vi "Teleop.vi"(6 "error in (no error)":errorcluster, 8 "Match Info":T1={"Autonomous Elapsed Seconds"=0.0, "TeleOp Elapsed Seconds"=0.0, "Disabled Elapsed Seconds"=0.0, "Visited Autonomous"=FALSE, "Visited TeleOp"=FALSE, "Visited Disabled"=FALSE, "Autonomous Settings"={"Autonomous Style"=enum."Independent", "VI Refnum"=refnum}}, 9 "Call Context":T2) -> (0 "error out":errorcluster, 1 "Throttle":dbl, 2 "Motors":dbl[](array[slide]) scale=-1.0..1.0)   [LabVIEW 2013]
doc: "This VI is called for each TeleOp packet received from the DS where the robot is not disabled. It is often used to read from the joysticks and update I/O or to update setpoints for timed control loops. It should complete and return within 20 milliseconds or it may miss DS packets."
uses:
  <vilib>/Rock Robotics/WPI/DriverStation/WPI_DriverStationDerivedRobotMode.ctl
  <vilib>/Rock Robotics/WPI/DriverStation/WPI_DriverStationMatch Info.ctl
  <vilib>/Rock Robotics/WPI/Relay/WPI_RelayValue.ctl
  Robot Global Data.vi
  <vilib>/Rock Robotics/WPI/RobotDrive/WPI_RobotDriveArcadeDrive_Standard(NoSaturation).vi
  <vilib>/Rock Robotics/WPI/Joystick/WPI_JoystickGetSetRefNum.vi
  <vilib>/Rock Robotics/WPI/RobotDrive/WPI_RobotDriveGetSetRefNum.vi
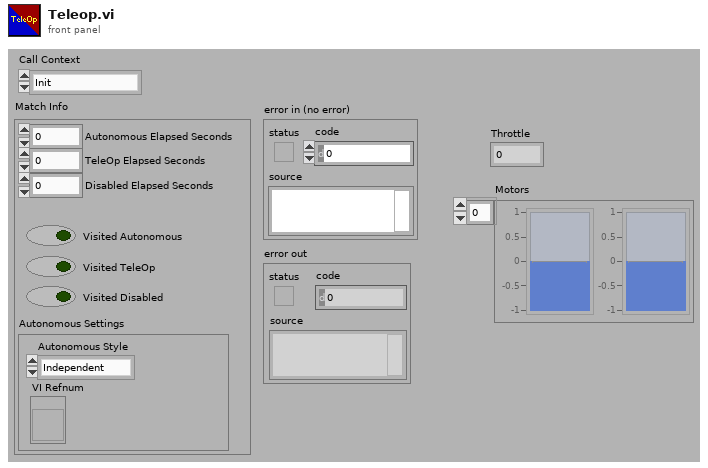
[diagram p1: front panel]
types:
  T1 = typedef "WPI_DriverStationMatch Info.ctl" = cluster{"Autonomous Elapsed Seconds":dbl, "TeleOp Elapsed Seconds":dbl, "Disabled Elapsed Seconds":dbl, "Visited Autonomous":bool, "Visited TeleOp":bool, "Visited Disabled":bool, "Autonomous Settings":cluster{"Autonomous Style":enum16{"Iterative", "Independent"}, "VI Refnum":refnum<vi>}}
  T2 = typedef "WPI_DriverStationDerivedRobotMode.ctl" = enum16{"Init", "Execute", "Stop"}
  T3 = typedef "WPI_JoystickDevRef.ctl" = cluster{"Device":T4}
  T4 = typedef "WPI_JoystickDeviceEnum.ctl" = enum16{"USB 1", "USB 2", "USB 3", "USB 4", "Kinect 1", "Kinect 2"}
  T5 = typedef "WPI_JoystickButtonState.ctl" = cluster{"Button 1":bool, "Button 2":bool, "Button 3":bool, "Button 4":bool, "Button 5":bool, "Button 6":bool, "Button 7":bool, "Button 8":bool, "Button 9":bool, "Button 10":bool, "Button 11":bool, "Button 12":bool}
  T6 = cluster{"axis 1 (x)":dbl, "axis 2 (y)":dbl, "axis 3 (throttle)":dbl, "axis 4":dbl, "axis 5":dbl, "axis 6":dbl}
  T7 = typedef "WPI_RelayValue.ctl" = enum16{"Off", "On", "Forward", "Reverse"}
  T8 = typedef "WPI_RobotDriveDevRef.ctl" = cluster{"DevStatus":errorcluster, "Motors[]":T9[], "Square Inputs":bool, "Max Output":dbl, "Isochronous":bool}
  T9 = typedef "WPI_MotorControlDeviceRef.ctl" = cluster{"DeviceStatus":errorcluster, "Type":enum16{"PWM", "CAN"}, "PWM":cluster{"Digital Module":T10, "PWM Channel":T11, "DeadBand":T12}, "CAN":cluster{"Device Number":u8, "Control Mode":T13, "Semaphore":T14, "Max Vout":dbl}, "Invert":bool, "TransformRef":T15, "InvTransformRef":T15}
  T10 = typedef "FPGA_TypedefDigitalModule.ctl" = enum16{"Digital Module 1", "Digital Module 2"}
  T11 = typedef "FPGA_DIOPWMChannel.ctl" = enum8{"PWM 1", "PWM 2", "PWM 3", "PWM 4", "PWM 5", "PWM 6", "PWM 7", "PWM 8", "PWM 9", "PWM 10", "Invalid"}
  T12 = typedef "WPI_PWMDeadband.ctl" = cluster{"Name":string, "maxPositivePwm":i32, "minPositivePwm":i32, "centerPwm":i32, "maxNegativePwm":i32, "minNegativePwm":i32, "angularRange":u16}
  T13 = typedef "WPI_CANJaguar_ControlMode.ctl" = enum8{"Percent VBus", "Current", "Speed", "Position", "Voltage"}
  T14 = typedef "Semaphore RefNum" = refnum<k1>
  T15 = typedef "WPI_PWMTransform_ConPane.ctl" = refnum<vi>
  T16 = typedef "WPI_RelayDevRef.ctl" = cluster{"DevStatus":errorcluster, "Relay Channel":T17, "Digital Module":T10, "Relay Direction":T18}
  T17 = typedef "FPGA_DIORelayChannel.ctl" = enum8{"Relay 1", "Relay 2", "Relay 3", "Relay 4", "Relay 5", "Relay 6", "Relay 7", "Relay 8", "Invalid"}
  T18 = typedef "WPI_RelayDirection.ctl" = enum16{"Both directions", "Forward only", "Reverse only"}
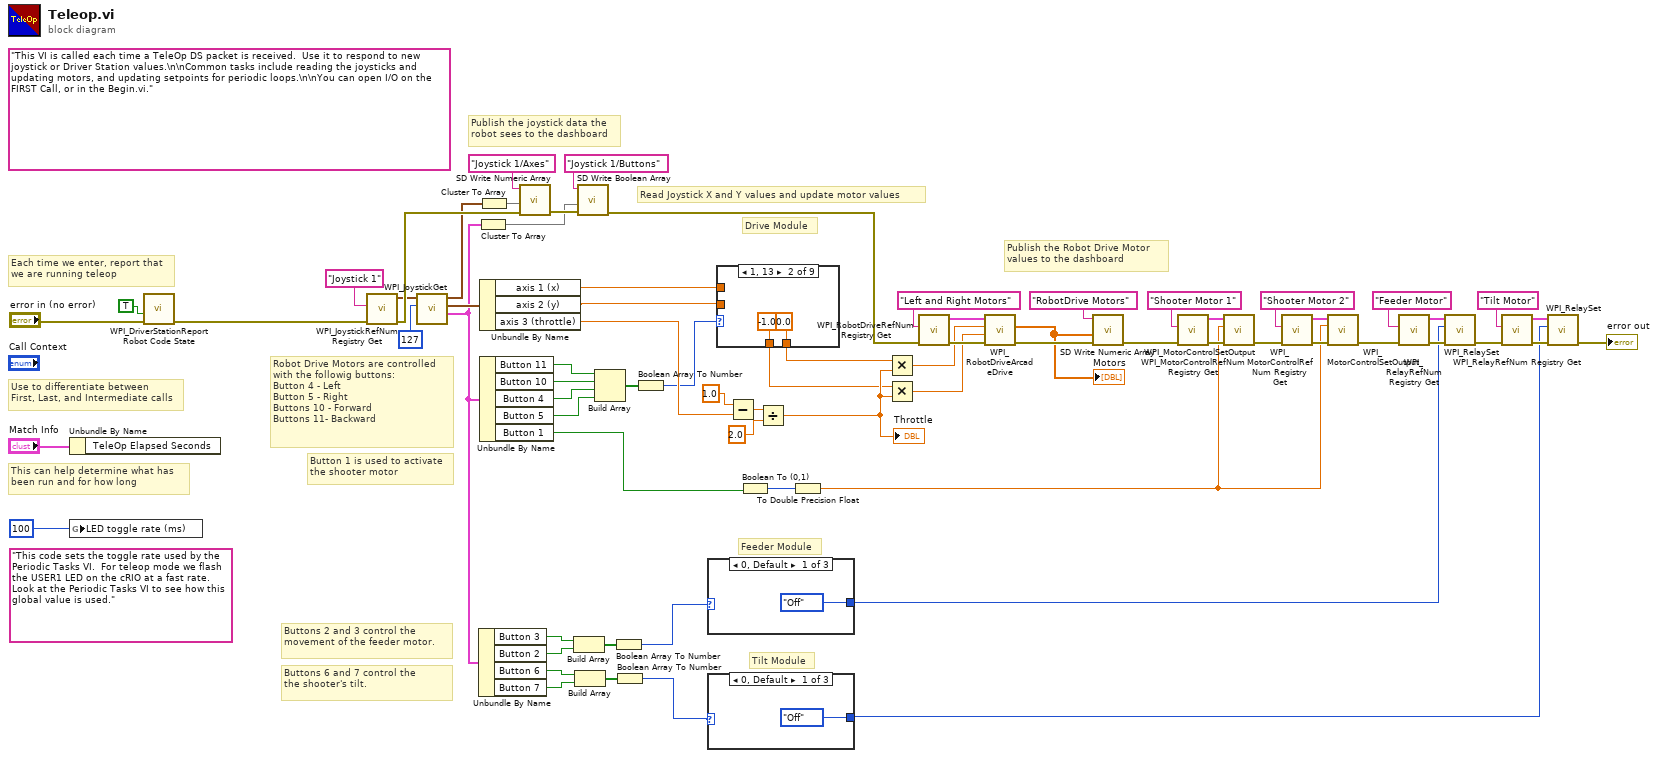
[diagram p0: block diagram]
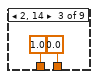
[diagram p3: hidden frame]
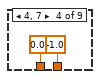
[diagram p4: hidden frame]
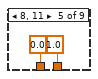
[diagram p5: hidden frame]
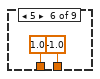
[diagram p6: hidden frame]
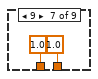
[diagram p7: hidden frame]
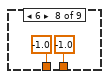
[diagram p8: hidden frame]
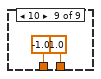
[diagram p9: hidden frame]
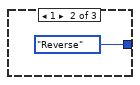
[diagram p10: hidden frame]
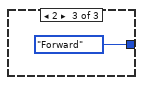
[diagram p11: hidden frame]
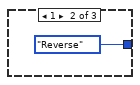
[diagram p12: hidden frame]
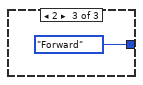
[diagram p13: hidden frame]
diagram:
  (unwired) "This code sets the toggle rate used by the Periodic Tasks VI.  For teleop mode we flash the USER1 LED on the cRIO at a fast rate.  Look at the Periodic Tasks VI to see how this global value is used."
  (unwired) "This VI is called each time a TeleOp DS packet is received.  Use it to respond to new joystick or Driver Station values.\n\nCommon tasks include reading the joysticks and updating motors, and updating setpoints for periodic loops.\n\nYou can open I/O on the FIRST Call, or in the Begin.vi."
  # "Buttons 6 and 7 control the\nthe shooter's tilt."
  # "Buttons 2 and 3 control the\nmovement of the feeder motor."
  # "Feeder Module"
  # "Tilt Module"
  # "Drive Module"
  # "Robot Drive Motors are controlled\nwith the followig buttons:\nButton 4 - Left\nButton 5 - Right\nButtons 10 - Forward\nButtons 11- Backward"
  # "Button 1 is used to activate\nthe shooter motor"
  # "Publish the Robot Drive Motor\nvalues to the dashboard"
  # "Read Joystick X and Y values and update motor values"
  # "Publish the joystick data the\nrobot sees to the dashboard"
  # "Each time we enter, report that\nwe are running teleop"
  # "Use to differentiate between\nFirst, Last, and Intermediate calls"
  # "This can help determine what has\nbeen run and for how long"
  n1 = Unbundle By Name("Match Info") -> ()  [unwired: 1 out]
  n2 = global write "Robot Global Data.vi" "LED toggle rate (ms)"(u32 100 ("LED ms toggle rate")) -> ()
  n3 = call <vilib>:"WPI_DriverStationReport Robot Code State.vi"("error in (no error)"="error in (no error)", "TeleOp"=TRUE ("Autonomous")) -> ("error out"=w43:errorcluster)  [unwired: 9 in]
  n4 = call <vilib>:"WPI_JoystickRefNum Registry Get.vi"("error in (no error)"=w43, "refnum name"="Joystick 1") -> ("error out"=w44:errorcluster, "JoystickDevRef"=w37:T3)  [unwired: 8 out]
  n5 = call <vilib>:"WPI_JoystickGet.vi"("Scaler"=i8 127, "JoystickDevRef"=w37) -> ("Buttons"=w34:T5, "Axes"=w51:T6, "JoystickDevRef"=w38:T3)  [unwired: 3 in]
  n6 = Cluster To Array(cluster=w34) -> (array=w39:bool[])
  n7 = Cluster To Array(cluster=w38) -> (array=w64:T4[])
  n8 = Unbundle By Name(w34) -> ("Button 3"=w20:bool, "Button 2"=w21:bool, "Button 6"=w59:bool, "Button 7"=w58:bool)
  n9 = Unbundle By Name(w51) -> ("axis 1 (x)"=w2:dbl, "axis 2 (y)"=w1:dbl, "axis 3 (throttle)"=w50:dbl)
  n10 = Unbundle By Name(w34) -> ("Button 11"=w55:bool, "Button 10"=w56:bool, "Button 4"=w36:bool, "Button 5"=w35:bool, "Button 1"=w7:bool)
  n11 = call <vilib>:"SD Write Numeric Array.vi"("error in"=w44, "Numeric Array"=w64, "Name"="Joystick 1/Axes") -> ("error out"=w42:errorcluster)  [unwired: 7 in, 1 out]
  n12 = Build Array(w20, w21) -> (w22:bool[])
  n13 = Build Array(w59, w58) -> (w57:bool[])
  n14 = call <vilib>:"SD Write Boolean Array.vi"("error in"=w42, "Boolean Array"=w39, "Name"="Joystick 1/Buttons") -> ("error out"=w41:errorcluster)  [unwired: 7 in, 1 out]
  n15 = Build Array(w55, w56, w36, w35) -> (w54:bool[])
  n16 = Boolean Array To Number(Boolean array=w22) -> (number=w19:u32)
  n17 = Boolean Array To Number(Boolean array=w57) -> (number=w11:u32)
  n18 = Boolean Array To Number(Boolean array=w54) -> (number=w3:u32)
  n19 = case shown="0, Default" w19 {
    tunnel: [WPI_RelayValue."Off" ("RelayValue") WPI_RelayValue."Reverse" ("RelayValue") WPI_RelayValue."Forward" ("RelayValue")] -> w12
    frame 0, Default {
    }
    frame 1 {
    }
    frame 2 {
    }
  }
  n20 = case shown="0, Default" w11 {
    tunnel: [WPI_RelayValue."Off" ("RelayValue") WPI_RelayValue."Reverse" ("RelayValue") WPI_RelayValue."Forward" ("RelayValue")] -> w10
    frame 0, Default {
    }
    frame 1 {
    }
    frame 2 {
    }
  }
  n21 = case shown="1, 13" w3 {
    tunnel: w2 -> [w79 _ _ _ _ _ _ _ _]
    tunnel: w1 -> [w78 _ _ _ _ _ _ _ _]
    tunnel: [w79 0.0 ("axis 1 (x)") 0.0 ("axis 1 (x)") -1.0 ("axis 1 (x)") 1.0 ("axis 1 (x)") -1.0 ("axis 1 (x)") 1.0 ("axis 1 (x)") -1.0 ("axis 1 (x)") 1.0 ("axis 1 (x)")] -> w5
    tunnel: [w78 -1.0 ("axis 2 (y)") 1.0 ("axis 2 (y)") 0.0 ("axis 2 (y)") 0.0 ("axis 2 (y)") 1.0 ("axis 2 (y)") 1.0 ("axis 2 (y)") -1.0 ("axis 2 (y)") -1.0 ("axis 2 (y)")] -> w4
    frame 0, Default {
    }
    frame 1, 13 {
    }
    frame 2, 14 {
    }
    frame 4, 7 {
    }
    frame 8, 11 {
    }
    frame 5 {
    }
    frame 9 {
    }
    frame 6 {
    }
    frame 10 {
    }
  }
  n22 = Subtract(x=1.0, y=w50) -> (x-y=w23:dbl)
  n23 = Boolean To (0,1)(Boolean=w7) -> (0, 1=w8:i16)
  n24 = Divide(x=w23, y=2.0) -> (x/y=w60:dbl)
  "Throttle" <- w60
  n25 = To Double Precision Float(number=w8) -> (double precision float=w6:dbl)
  n26 = Multiply(x=w5, y=w60) -> (x*y=w32:dbl)
  n27 = Multiply(x=w4, y=w60) -> (x*y=w31:dbl)
  n28 = call <vilib>:"WPI_RobotDriveRefNum Registry Get.vi"("error in (no error)"=w41, "refnum name"="Left and Right Motors") -> ("error out"=w47:errorcluster, "RobotDriveDevRef"=w61:T8)  [unwired: 8 out]
  n29 = call-poly <vilib>:"WPI_RobotDriveArcadeDrive.vi"("error in (no error)"=w47, "Y axis value"=w31, "X axis value"=w32, "RobotDriveDevRef"=w61) -> ("error out"=w40:errorcluster, "Motor Values"=w13:dbl[])  [unwired: 5 in, 1 out]
  "Motors" <- w13
  n30 = call <vilib>:"SD Write Numeric Array.vi"("error in"=w40, "Numeric Array"=w13, "Name"="RobotDrive Motors") -> ("error out"=w45:errorcluster)  [unwired: 7 in, 1 out]
  n31 = call <vilib>:"WPI_MotorControlRefNum Registry Get.vi"("error in (no error)"=w45, "refnum name"="Shooter Motor 1") -> ("error out"=w46:errorcluster, "MotorControlDevRef"=w68:T9)  [unwired: 8 in]
  n32 = call <vilib>:"WPI_MotorControlSetOutput.vi"("error in (no error)"=w46, "Output"=w6, "MotorControlDevRef"=w68) -> ("error out"=w16:errorcluster)  [unwired: 6 in, 2 out]
  n33 = call <vilib>:"WPI_MotorControlRefNum Registry Get.vi"("error in (no error)"=w16, "refnum name"="Shooter Motor 2") -> ("error out"=w15:errorcluster, "MotorControlDevRef"=w17:T9)  [unwired: 8 in]
  n34 = call <vilib>:"WPI_MotorControlSetOutput.vi"("error in (no error)"=w15, "Output"=w6, "MotorControlDevRef"=w17) -> ("error out"=w14:errorcluster)  [unwired: 6 in, 2 out]
  n35 = call <vilib>:"WPI_RelayRefNum Registry Get.vi"("error in (no error)"=w14, "refnum name"="Feeder Motor") -> ("error out"=w29:errorcluster, "RelayDevRef"=w27:T16)  [unwired: 8 in]
  n36 = call <vilib>:"WPI_RelaySet.vi"("error in (no error)"=w29, "RelayValue"=w12, "RelayDevRef"=w27) -> ("error out"=w26:errorcluster)  [unwired: 7 in, 1 out]
  n37 = call <vilib>:"WPI_RelayRefNum Registry Get.vi"("error in (no error)"=w26, "refnum name"="Tilt Motor") -> ("error out"=w49:errorcluster, "RelayDevRef"=w53:T16)  [unwired: 8 in]
  n38 = call <vilib>:"WPI_RelaySet.vi"("error in (no error)"=w49, "RelayValue"=w10, "RelayDevRef"=w53) -> ("error out"=→"error out":errorcluster)  [unwired: 7 in, 1 out]
